vi "DCMotortest.vi"(7 "Reset":bool, 8 "error in":errorcluster, 10 "PWM":dbl) -> (0 "error out":errorcluster, 2 "Encoder":dbl)   [LabVIEW 2019]
uses:
  KNRm_ReMi_OS5.lvlibp
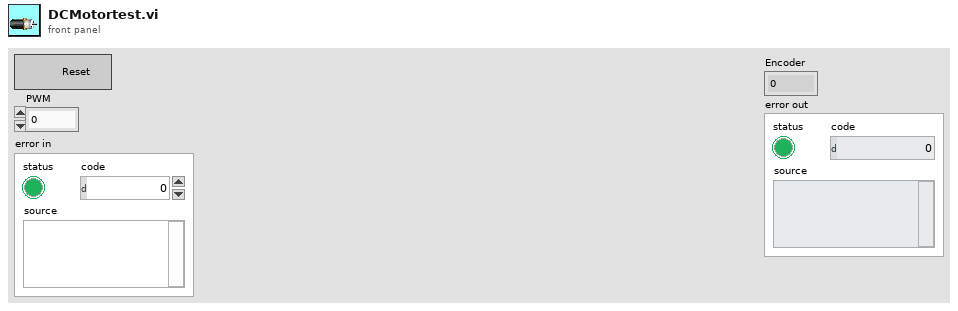
[diagram p1: front panel]
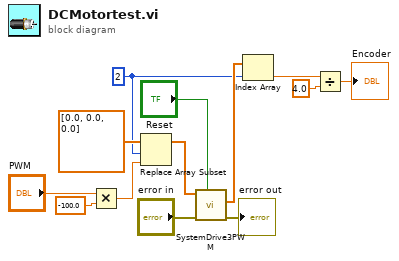
[diagram p0: block diagram]
diagram:
  w9 = 2 ("index")
  n1 = Multiply(x="PWM", y=-100.0) -> (x*y=w5:dbl)
  n2 = Replace Array Subset(array=dbl[] [0.0, 0.0, 0.0] ("3xMotorSpeed(PWM%)"), new element=w5, index=w9) -> (w11:dbl[])
  n3 = call "SystemDrive3PWM.vi"("Reset"="Reset", "error in"="error in", "3xMotorSpeed(PWM%)"=w11) -> ("error out"=→"error out":errorcluster, "ENC (deg)"=w10:dbl[])  [unwired: 7 in]
  n4 = Index Array(array=w10, index=w9) -> (element=w1:dbl)
  n5 = Divide(x=w1, y=4.0) -> (x/y=→"Encoder":dbl)
